vi "0703  Motor Drive System_V2.vi"() -> ()   [LabVIEW 2018]
uses:
  <vilib>/Instr/_visa.llb/VISA Configure Serial Port (Instr).vi
panel:
  in  "停止":bool
  in  "关闭程序：":bool
  out "错误输出":errorcluster
  in  "开/关 VISA：":bool
  in  "VISA resource name":refnum<visa-resource-name> caption="VISA资源名称："
  in  "baud rate (9600)":u32=9600 caption="波特率："
  in  "脉冲频率":dbl(knob) scale=10.0..400.0
  in  "顺         逆":bool
  in  "旋转角度":u16
  in  "执行":bool
  # "电机驱动系统"
  # "Motor_Drive_System_V2\nBy Liu Guangxin\n2020.07.03"
  # "操作面板"
  # "VISA参数配置"
  # "°"
  # "Hz"
  # "顺            逆"
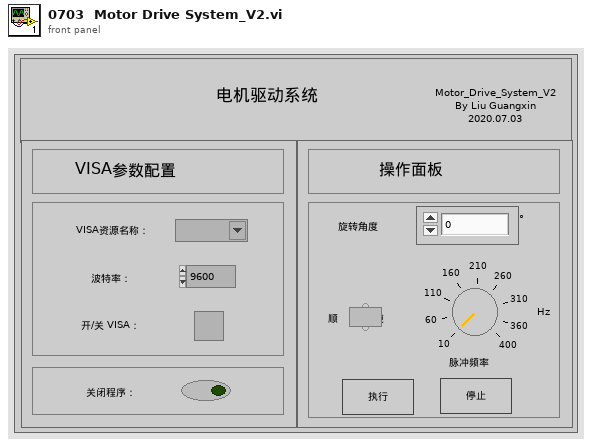
[diagram p1: front panel]
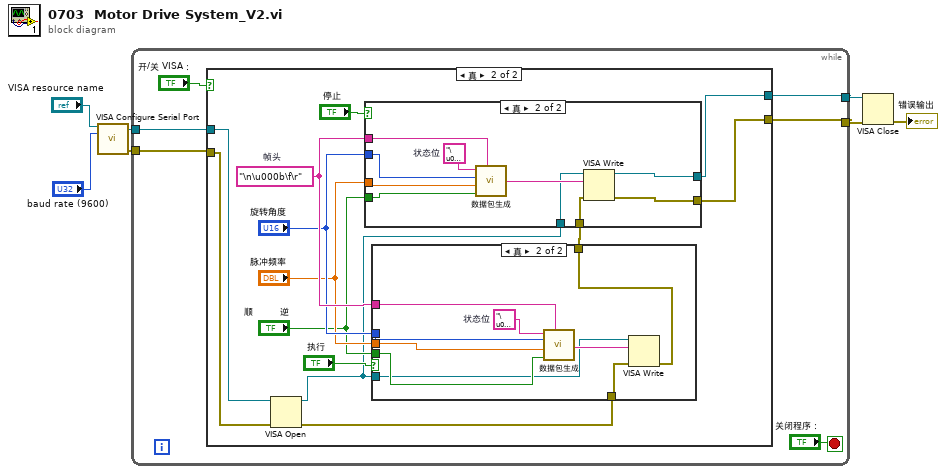
[diagram p0: block diagram]
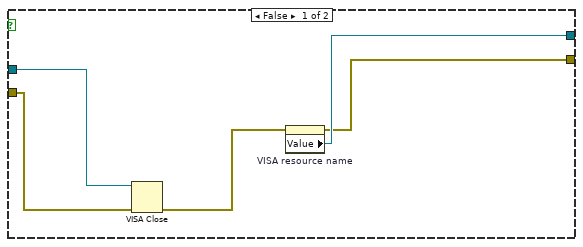
[diagram p2: hidden frame]
diagram:
  n1 = call-poly "VISA Configure Serial Port"("VISA resource name"="VISA resource name", "baud rate (9600)"="baud rate (9600)") -> ("VISA resource name out"=w3:refnum<visa-resource-name>, "error out"=w4:errorcluster)  [unwired: 12 in]
  n2 = while {
    tunnel: w4 -> [w11]
    tunnel: w3 -> [w8]
    tunnel: [w9] -> w2
    tunnel: [w10] -> w1
    stop <- "关闭程序：" stop-if-true
    n3 = case shown="真" "开/关 VISA：" {
      tunnel: w11 -> [w18 w30]
      tunnel: [w15 w19] -> w10
      tunnel: [w17 w29] -> w9
      tunnel: w8 -> [w14 w28]
      frame False {
        n4 = VISA Close(VISA resource name=w14, error in (no error)=w18) -> (error out=w16:errorcluster)
        n5 = property on="VISA resource name" class="VISAName"(error in=w16) -> (error out=w15:errorcluster, "Value"=w17:refnum<visa-resource-name>)  [unwired: 1 in, 1 out]
      }
      frame True {
        w26 = "\n\u000b\f\r"  # 帧头
        n6 = VISA Open(error in (no error)=w30, VISA resource name=w28) -> (VISA resource name=w21:refnum<visa-resource-name>, error out=w22:errorcluster)  [unwired: 3 in]
        n7 = case shown="真" "执行" {
          tunnel: w22 -> [w32 w39]
          tunnel: w26 -> [_ w38]
          tunnel: "旋转角度" -> [_ w37]
          tunnel: "脉冲频率" -> [_ w36]
          tunnel: "顺         逆" -> [_ w35]
          tunnel: w21 -> [_ w34]
          tunnel: [w32 w33] -> w20
          frame False {
          }
          frame True {
            w41 = "\u0000"  # 状态位
            n8 = call "数据包生成.vi"("状态："=w41, "旋转角度："=w37, "脉冲频率："=w36, "旋转方向："=w35, "帧头："=w38) -> ("数据包"=w40:string)
            n9 = VISA Write(VISA resource name=w34, write buffer=w40, error in (no error)=w39) -> (error out=w33:errorcluster)  [unwired: 2 out]
          }
        }
        n10 = case shown="真" "停止" {
          tunnel: [w42 w51] -> w19
          tunnel: [w43 w50] -> w29
          tunnel: w26 -> [_ w49]
          tunnel: "旋转角度" -> [_ w48]
          tunnel: "脉冲频率" -> [_ w47]
          tunnel: "顺         逆" -> [_ w46]
          tunnel: w21 -> [w43 w45]
          tunnel: w20 -> [w42 w44]
          frame False {
          }
          frame True {
            w53 = "\u0001"  # 状态位
            n11 = call "数据包生成.vi"("状态："=w53, "旋转角度："=w48, "脉冲频率："=w47, "旋转方向："=w46, "帧头："=w49) -> ("数据包"=w52:string)
            n12 = VISA Write(VISA resource name=w45, write buffer=w52, error in (no error)=w44) -> (VISA resource name out=w50:refnum<visa-resource-name>, error out=w51:errorcluster)  [unwired: 1 out]
          }
        }
      }
    }
  }
  n13 = VISA Close(VISA resource name=w2, error in (no error)=w1) -> (error out=→"错误输出":errorcluster)
